vi "FIFORequests.vi"(1 "New One":T1, 2 "data out":string, 3 "Requests In":T2(array[cluster])) -> (0 "Requests Out":T2(array[cluster]))   [LabVIEW 2010]
uses:
  _ROSDefinition.vi
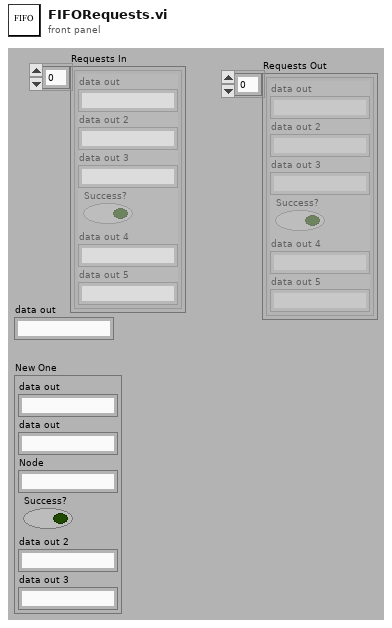
[diagram p1: front panel]
types:
  T1 = cluster{"data out":string, "data out":string, "Node":string, "Success?":bool, "data out 2":string, "data out 3":string}
  T2 = cluster{"data out":string, "data out 2":string, "data out 3":string, "Success?":bool, "data out 4":string, "data out 5":string}[]
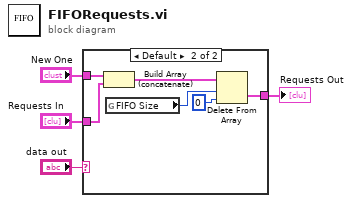
[diagram p0: block diagram]
diagram:
  n1 = case shown="Default" "data out" {
    tunnel: "New One" -> [_ w8]
    tunnel: "Requests In" -> [w5 w9]
    tunnel: [w5 w10] -> w3
    frame "" {
    }
    frame Default {
      n2 = Build Array (concatenate)(w8, w9) -> (w11:T2)
      n3 = global read "_ROSDefinition.vi" "FIFO Size"() -> (w6:i32)
      n4 = Delete From Array(array=w11, length=w6, index=0) -> (deleted portion=w10:T2)  [unwired: 1 out]
    }
  }
  "Requests Out" <- w3
